vi "audio2.vi"(11 "queue out":refnum<queue>) -> ()   [LabVIEW 2010]
uses:
  <vilib>/sound2/lvsound2.llb/Sampling Mode.ctl
  <vilib>/sound2/lvsound2.llb/Sound Data Format.ctl
  <vilib>/sound2/lvsound2.llb/Sound Output Write (DBL Single).vi
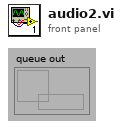
[diagram p1: front panel]
types:
  T1 = typedef "Sound Data Format.ctl" = cluster{"sample rate (S/s)":dbl, "number of channels":i32, "bits per sample":i32}
  T2 = typedef "Sampling Mode.ctl" = i32
  T3 = typedef "Sound Output Task ID.ctl" = u32
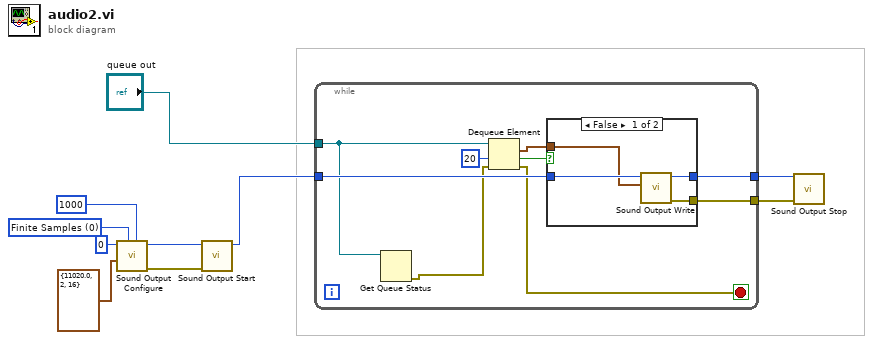
[diagram p0: block diagram]
diagram:
  w10 = T2 0 items=["Finite Samples", "Continuous Samples"] ("sample mode")
  n1 = call <vilib>:"Sound Output Configure.vi"("number of samples/ch"=1000, "sample mode"=w10, "sound format"=T1 {"sample rate (S/s)"=11020.0, "number of channels"=2, "bits per sample"=16}, "device ID"=u32 0) -> ("error out"=w6:errorcluster, "task ID"=w7:T3)  [unwired: 6 in]
  n2 = call <vilib>:"Sound Output Start.vi"("error in (no error)"=w6, "task ID"=w7) -> ("task ID out"=w5:T3)  [unwired: 8 in, 1 out]
  n3 = while {
    tunnel: "queue out" -> [w15]
    tunnel: w5 -> [w16]
    tunnel: [w12] -> w4
    tunnel: [w11] -> w3
    stop <- w13 stop-if-true
    n4 = Get Queue Status(queue=w15) -> (error out=w14:errorcluster)  [unwired: 2 in, 7 out]
    n5 = Dequeue Element(queue=w15, timeout in ms (-1)=20, error in (no error)=w14) -> (element=w17:waveform(dbl), timed out?=w18:bool, error out=w13:errorcluster)  [unwired: 1 out]
    n6 = case shown="False" w18 {
      tunnel: w17 -> [w22 _]
      tunnel: w16 -> [w23 w24]
      tunnel: [w21 w24] -> w12
      tunnel: [w20 _] -> w11
      frame False {
        n7 = call-poly <vilib>:"Sound Output Write.vi"("data"=w22, "task ID"=w23) -> ("error out"=w20:errorcluster, "task ID out"=w21:T3)  [unwired: 8 in]
      }
      frame True {
      }
    }
  }
  n8 = call <vilib>:"Sound Output Stop.vi"("error in (no error)"=w3, "task ID"=w4) -> ()  [unwired: 8 in, 2 out]
